vi "CODMn质控流程 (子VI).vi"(9 "CODMn量程切换":enum32{"H", "L", "AUTO"}(ring)=enum."AUTO", 10 "CODMn":bool) -> (3 "布尔":bool)   [LabVIEW 2016, in "质控单元.lvlib"]
panel:
  out "CODMn中断报警":bool
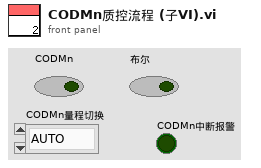
[diagram p1: front panel]
types:
  T1 = enum16{"待机", "启动水样测量", "水样测量中", "启动加标", "启动加标回收", "加标回收测量中", "结束"}
  T2 = cluster{"测量模式":enum16{"水样测量", "标样核查", "零点核查", "跨度核查", "空白测试", "加标回收", "平行样", "校零", "校标"}}
  T3 = enum16{"空闲", "水样测试", "标样核查", "零点核查", "跨度核查", "空白测试", "平行样测试", "质控样", "空白校准", "标样校准", "加标回收"}
  T4 = cluster{"量程":dbl, "检出限":dbl, "加标前水样浓度":dbl, "加标后水样浓度":dbl, "加标水杯定容体积":dbl, "加标母液浓度":dbl, "加标体积":dbl, "加标回收率":dbl}
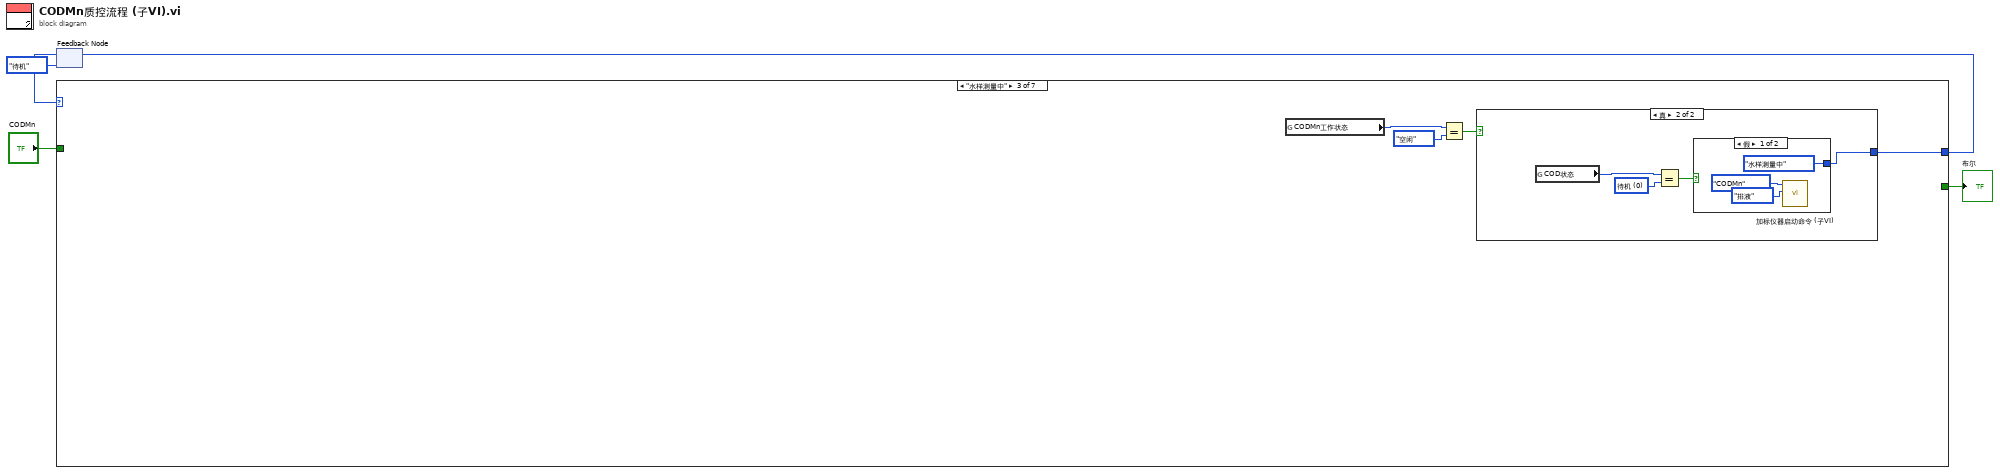
[diagram p0: block diagram]
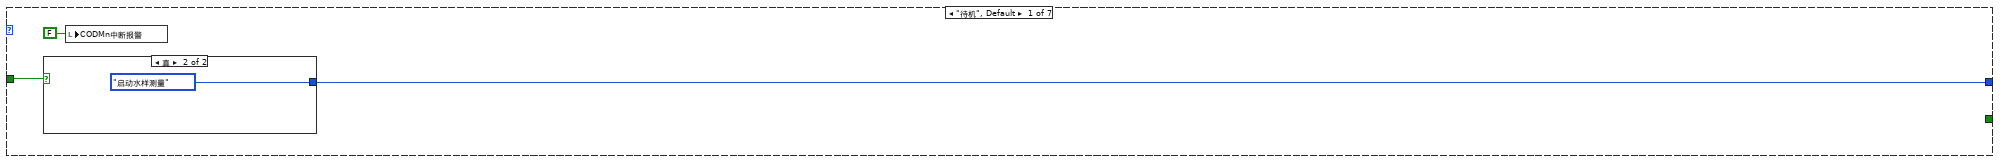
[diagram p2: hidden frame]
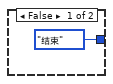
[diagram p3: hidden frame]
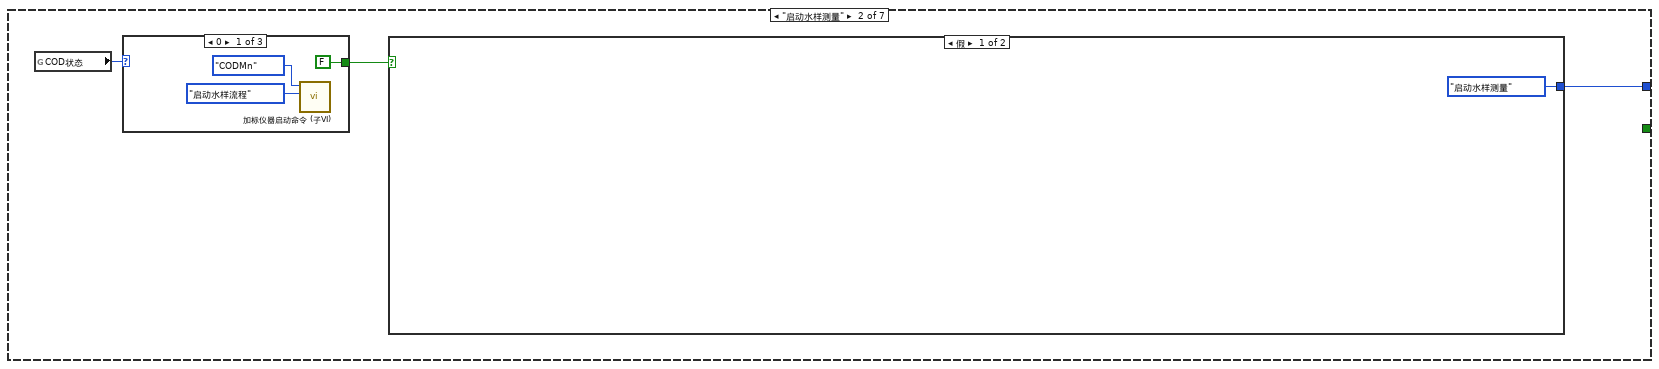
[diagram p4: hidden frame]
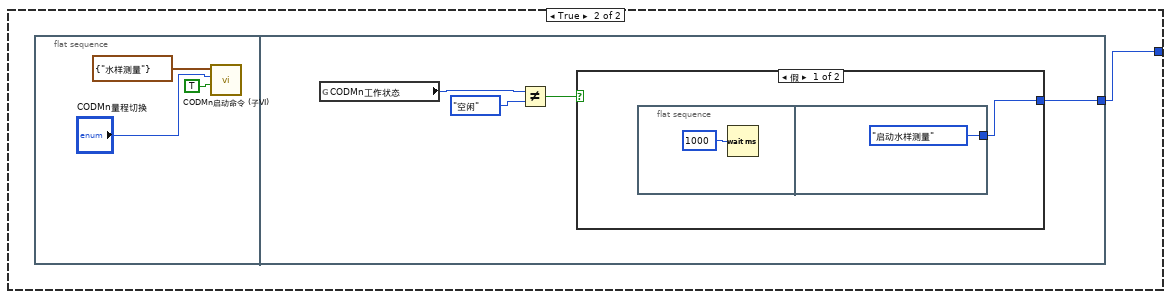
[diagram p5: hidden frame]
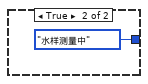
[diagram p6: hidden frame]
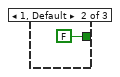
[diagram p7: hidden frame]
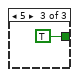
[diagram p8: hidden frame]
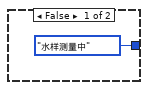
[diagram p9: hidden frame]
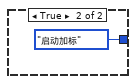
[diagram p10: hidden frame]
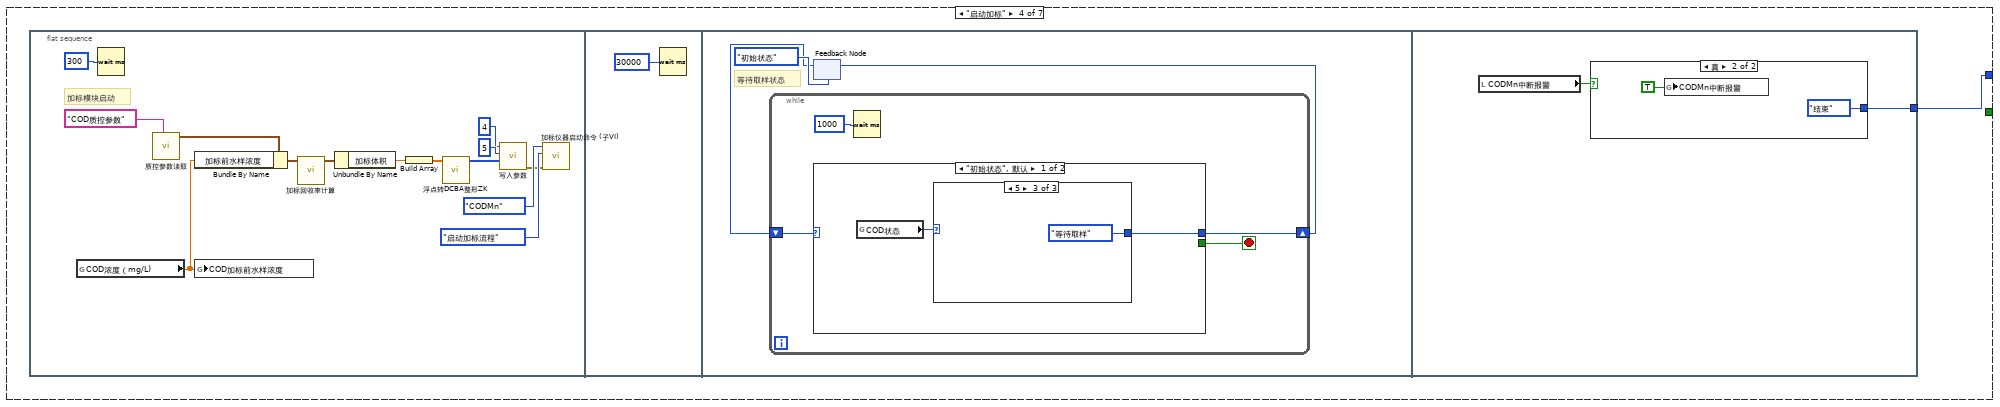
[diagram p11: hidden frame]
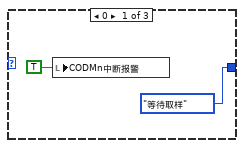
[diagram p12: hidden frame]
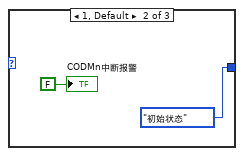
[diagram p13: hidden frame]
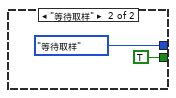
[diagram p14: hidden frame]
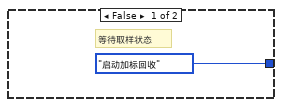
[diagram p15: hidden frame]
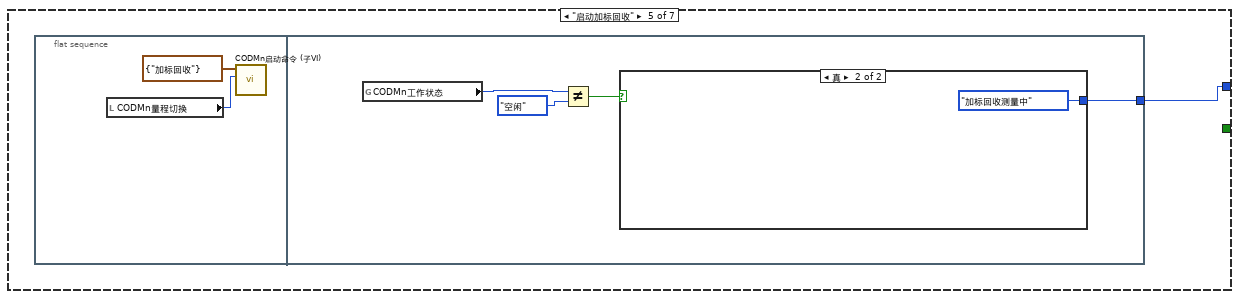
[diagram p16: hidden frame]
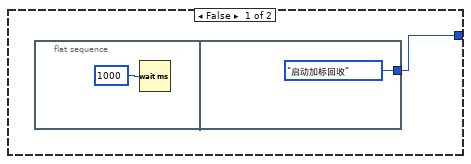
[diagram p17: hidden frame]
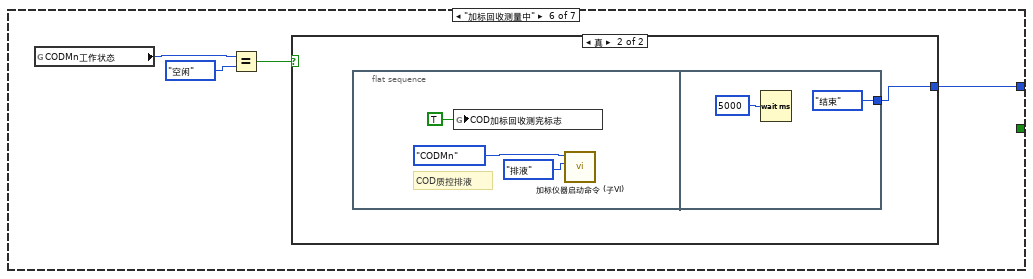
[diagram p18: hidden frame]
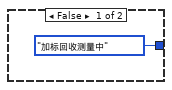
[diagram p19: hidden frame]
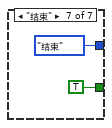
[diagram p20: hidden frame]
diagram:
  n1 = feedback #1(T1."待机") -> (w3:T1)
  n2 = case shown="\"水样测量中\"" w3 {
    tunnel: [w8 w13 w35 w45 w82 w96 T1."结束"] -> w4
    tunnel: [_ _ _ _ _ _ TRUE] -> w2
    tunnel: "CODMn" -> [w7 _ _ _ _ _ _]
    frame "待机", Default {
      n3 = case shown="真" w7 {
        tunnel: [T1."结束" T1."启动水样测量"] -> w8
        frame False {
        }
        frame True {
        }
      }
      n4 = local write "CODMn中断报警"(FALSE ("CODMn中断报警")) -> ()
    }
    frame "启动水样测量" {
      n5 = global read "加标回收状态全局变量.vi" "COD状态"() -> (w12:u16)
      n6 = case shown="0" w12 {
        tunnel: [FALSE ("s") FALSE ("s") TRUE ("s")] -> w11
        frame 0 {
          n7 = call "加标仪器启动命令 (子VI).vi"("启动命令"=enum16{"启动水样流程", "启动加标流程", "排液", "停止"}."启动水样流程", "仪器"=enum16{"", "氨氮", "总磷", "总氮", "CODMn", "CODCr"}."CODMn") -> ()  [unwired: 9 in, 1 out]
        }
        frame 1, Default {
        }
        frame 5 {
        }
      }
      n8 = case shown="假" w11 {
        tunnel: [T1."启动水样测量" w15] -> w13
        frame False {
        }
        frame True {
          n9 = flat-sequence {
            tunnel: [w22] -> w15
            frame #0 {
              n10 = call "CODMn启动命令 (子VI).vi"("强制切换"=TRUE, "CODMn量程切换"="CODMn量程切换", "启动测量模式"=T2 {"测量模式"=enum."水样测量"}) -> ()  [unwired: 8 in, 1 out]
            }
            frame #1 {
              n11 = global read "与CODMn交互全局.vi" "CODMn工作状态"() -> (w21:T3)
              n12 = Not Equal?(x=w21, y=T3."空闲") -> (x != y?=w19:bool)
              n13 = case shown="假" w19 {
                tunnel: [w23 T1."水样测量中"] -> w22
                frame False {
                  n14 = flat-sequence {
                    tunnel: [T1."启动水样测量"] -> w23
                    frame #0 {
                      n15 = Wait (ms)(milliseconds to wait=u32 1000 ("等待时间（毫秒）")) -> ()  [unwired: 1 out]
                    }
                    frame #1 {
                    }
                  }
                }
                frame True {
                }
              }
            }
          }
        }
      }
    }
    frame "水样测量中" {
      n16 = global read "与CODMn交互全局.vi" "CODMn工作状态"() -> (w34:T3)
      n17 = Equal?(x=w34, y=T3."空闲") -> (x = y?=w32:bool)
      n18 = case shown="真" w32 {
        tunnel: [T1."水样测量中" w40] -> w35
        frame False {
        }
        frame True {
          w38 = u16 0 items=["待机", "润洗", "进样", "进样完成", "柱塞泵加标", "等待取液", "排液"] ("COD状态")
          n19 = global read "加标回收状态全局变量.vi" "COD状态"() -> (w39:u16)
          n20 = Equal?(x=w39, y=w38) -> (x = y?=w37:bool)
          n21 = case shown="假" w37 {
            tunnel: [T1."水样测量中" T1."启动加标"] -> w40
            frame False {
              n22 = call "加标仪器启动命令 (子VI).vi"("启动命令"=enum16{"启动水样流程", "启动加标流程", "排液", "停止"}."排液", "仪器"=enum16{"", "氨氮", "总磷", "总氮", "CODMn", "CODCr"}."CODMn") -> ()  [unwired: 9 in, 1 out]
            }
            frame True {
            }
          }
        }
      }
    }
    frame "启动加标" {
      n23 = flat-sequence {
        tunnel: [w78] -> w45
        frame #0 {
          # "加标模块启动"
          n24 = global read "与CODMn交互全局.vi" "COD浓度（mg/L)"() -> (w53:dbl)
          n25 = Wait (ms)(milliseconds to wait=u32 300 ("等待时间（毫秒）")) -> ()  [unwired: 1 out]
          n26 = call "质控参数读取.vi"("section"="COD质控参数") -> ("参数"=w57:T4)  [unwired: 9 in, 1 out]
          n27 = Bundle By Name(cluster=w57, "加标前水样浓度"=w53) -> (w58:T4)
          n28 = global write "水样浓度全局.vi" "COD加标前水样浓度"(w53) -> ()
          n29 = call "加标回收率计算.vi"("参数"=w58) -> ("参数 out"=w56:T4)  [unwired: 10 in]
          n30 = Unbundle By Name(w56) -> ("加标体积"=w54:dbl)
          n31 = Build Array(w54) -> (w50:dbl[])
          n32 = call "浮点转DCBA整形ZK.vi"("浮点数"=w50) -> ("DCBA整形输出"=w49:u16[])  [unwired: 10 in]
          n33 = call "写入参数.vi"("values"=w49, "starting address"=u16 5, "Slave ID"=u16 4 ("value")) -> ("error out"=w46:errorcluster)  [unwired: 8 in]
          n34 = call "加标仪器启动命令 (子VI).vi"("Error in"=w46, "启动命令"=enum16{"启动水样流程", "启动加标流程", "排液", "停止"}."启动加标流程", "仪器"=enum16{"", "氨氮", "总磷", "总氮", "CODMn", "CODCr"}."CODMn") -> ()  [unwired: 8 in, 1 out]
        }
        frame #1 {
          n35 = Wait (ms)(milliseconds to wait=u32 30000 ("等待时间（毫秒）")) -> ()  [unwired: 1 out]
        }
        frame #2 {
          # "等待取样状态"
          n36 = feedback #2(enum16{"初始状态", "等待取样"}."初始状态") -> (w62:enum16{"初始状态", "等待取样"})
          n37 = while {
            shift-right: [w66] -> w61
            shift-left: w62 -> [w67]
            stop <- w65 stop-if-true
            n38 = case shown="\"初始状态\", 默认" w67 {
              tunnel: [w69 enum16{"初始状态", "等待取样"}."等待取样"] -> w66
              tunnel: [_ TRUE] -> w65
              frame "初始状态", Default {
                n39 = global read "加标回收状态全局变量.vi" "COD状态"() -> (w68:u16)
                n40 = case shown="5" w68 {
                  tunnel: [enum16{"初始状态", "等待取样"}."等待取样" enum16{"初始状态", "等待取样"}."初始状态" enum16{"初始状态", "等待取样"}."等待取样"] -> w69
                  frame 0 {
                    n41 = local write "CODMn中断报警"(TRUE ("氨氮中断报警")) -> ()
                  }
                  frame 1, Default {
                    "CODMn中断报警" <- FALSE ("总氮中断报警")
                  }
                  frame 5 {
                  }
                }
              }
              frame "等待取样" {
              }
            }
            n42 = Wait (ms)(milliseconds to wait=u32 1000 ("等待时间（毫秒）")) -> ()  [unwired: 1 out]
          }
          n43 = feedback-in #2(w61) -> ()
        }
        frame #3 {
          n44 = local read "CODMn中断报警"() -> (w77:bool)
          n45 = case shown="真" w77 {
            tunnel: [T1."启动加标回收" T1."结束"] -> w78
            frame False {
              # "等待取样状态"
            }
            frame True {
              n46 = global write "质控中断报警全局.vi" "CODMn中断报警"(TRUE ("CODMn中断报警")) -> ()
            }
          }
        }
      }
    }
    frame "启动加标回收" {
      n47 = flat-sequence {
        tunnel: [w88] -> w82
        frame #0 {
          n48 = local read "CODMn量程切换"() -> (w84:enum32{"H", "L", "AUTO"})
          n49 = call "CODMn启动命令 (子VI).vi"("CODMn量程切换"=w84, "启动测量模式"=T2 {"测量模式"=enum."加标回收"}) -> ()  [unwired: 9 in, 1 out]
        }
        frame #1 {
          n50 = global read "与CODMn交互全局.vi" "CODMn工作状态"() -> (w87:T3)
          n51 = Not Equal?(x=w87, y=T3."空闲") -> (x != y?=w85:bool)
          n52 = case shown="真" w85 {
            tunnel: [w89 T1."加标回收测量中"] -> w88
            frame False {
              n53 = flat-sequence {
                tunnel: [T1."启动加标回收"] -> w89
                frame #0 {
                  n54 = Wait (ms)(milliseconds to wait=u32 1000 ("等待时间（毫秒）")) -> ()  [unwired: 1 out]
                }
                frame #1 {
                }
              }
            }
            frame True {
            }
          }
        }
      }
    }
    frame "加标回收测量中" {
      n55 = global read "与CODMn交互全局.vi" "CODMn工作状态"() -> (w95:T3)
      n56 = Equal?(x=w95, y=T3."空闲") -> (x = y?=w93:bool)
      n57 = case shown="真" w93 {
        tunnel: [T1."加标回收测量中" w98] -> w96
        frame False {
        }
        frame True {
          n58 = flat-sequence {
            tunnel: [T1."结束"] -> w98
            frame #0 {
              # "COD质控排液"
              n59 = global write "质控测完标志全局 1.vi" "COD加标回收测完标志"(TRUE ("COD加标回收测完标志")) -> ()
              n60 = call "加标仪器启动命令 (子VI).vi"("启动命令"=enum16{"启动水样流程", "启动加标流程", "排液", "停止"}."排液", "仪器"=enum16{"", "氨氮", "总磷", "总氮", "CODMn", "CODCr"}."CODMn") -> ()  [unwired: 9 in, 1 out]
            }
            frame #1 {
              n61 = Wait (ms)(milliseconds to wait=u32 5000 ("等待时间（毫秒）")) -> ()  [unwired: 1 out]
            }
          }
        }
      }
    }
    frame "结束" {
    }
  }
  "布尔" <- w2
  n62 = feedback-in #1(w4) -> ()
